vi "Integration Reset.vi"(8 "error in (no error)":errorcluster, 11 "Yokogawa WT500 in":refnum<class "Yokogawa WT500.lvclass">) -> (0 "error out":errorcluster, 2 "VISA resource name":refnum<visa-resource-name>, 3 "Yokogawa WT500 out":refnum<class "Yokogawa WT500.lvclass">)   [LabVIEW 2013, in "Universal Power Meter.lvlib" / "Yokogawa WT500.lvlib" / "Yokogawa WT500.lvclass"]
uses:
  Yokogawa WT500.lvclass
  Universal Power Meter class/Universal Power Meter.lvclass
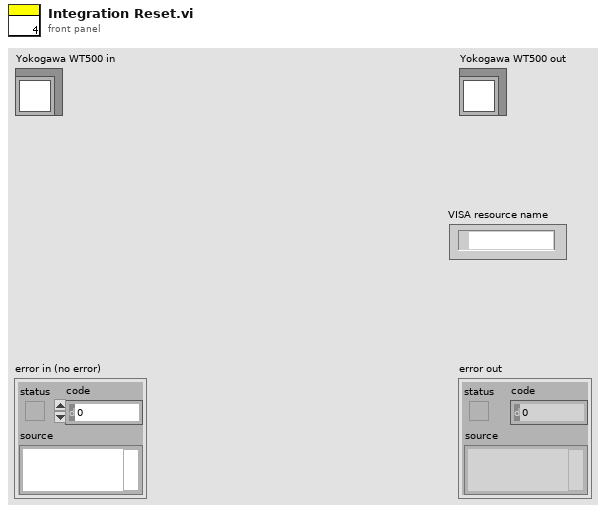
[diagram p1: front panel]
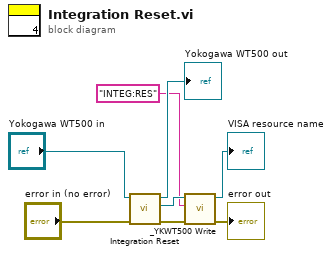
[diagram p0: block diagram]
diagram:
  n1 = call-parent "Integration Reset.vi"("error in (no error)"="error in (no error)", "Universal Power Meter in"="Yokogawa WT500 in") -> ("error out"=w3:errorcluster, "VISA resource name"=w5:refnum<visa-resource-name>, "Universal Power Meter out"=→"Yokogawa WT500 out":refnum<class "Yokogawa WT500.lvclass">)  [unwired: 7 in]
  n2 = call <instrlib>:"_YKWT500 Write.vi"("error in (no error)"=w3, "Write Data"="INTEG:RES", "VISA resource name"=w5) -> ("error out"=→"error out":errorcluster, "VISA resource name out"=→"VISA resource name":refnum<visa-resource-name>)  [unwired: 5 in, 2 out]
